vi "sendDefaultILCOutputs.vi"(8 "error in (no error)":errorcluster, 11 "Model in":refnum<class "Model.lvclass">) -> (0 "error out":errorcluster, 3 "Model out":refnum<class "Model.lvclass">)   [LabVIEW 2015, in "Model.lvclass"]
uses:
  Model.lvclass
  Typedefs/Actuate Settings.ctl
  Typedefs/ControlMode.ctl
  Model.lvclass/Model.ctl
  Actuator/IActuator/IActuator.lvclass
  <userlib>/Common/ILC/ILC/ILC.lvclass
  Typedefs/FAMTTypedefs.lvlib
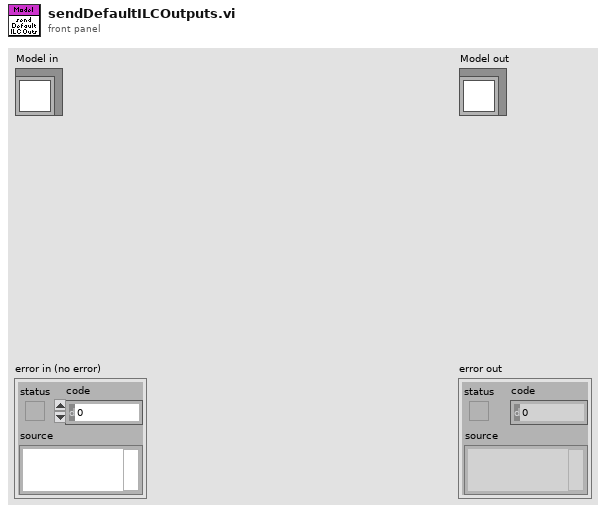
[diagram p1: front panel]
types:
  T1 = typedef "FAMTTypedefs.lvlib/ControlMode.ctl" = enum16{"PSV", "FCV", "Both"}
  T2 = typedef "FAMTTypedefs.lvlib/Actuate Settings.ctl" = cluster{"Control Mode":T1, "Control Value":dbl, "Measured Value":dbl[unit], "FCV Value":dbl}
  T3 = typedef "FAMTTypedefs.lvlib/Flow Control Settings.ctl" = cluster{"DAC Channel":u8, "ROT Bias":u8, "Minimum Voltage":dbl, "Maximum Voltage":dbl, "Off Value":dbl}
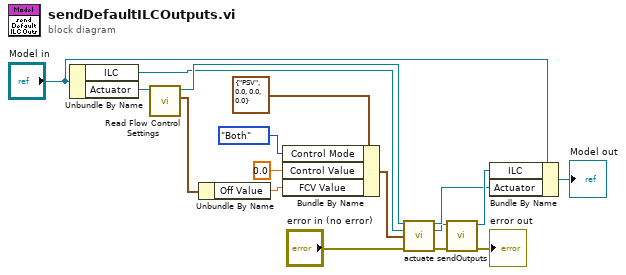
[diagram p0: block diagram]
diagram:
  n1 = Unbundle By Name("Model in") -> ("ILC"=w10:refnum<class "ILC.lvclass">, "Actuator"=w1:refnum<class "IActuator.lvclass">)
  n2 = call-dynamic "Read Flow Control Settings.vi"("IActuator in"=w1) -> ("Flow Control Settings"=w14:T3, "IActuator out"=w13:refnum<class "IActuator.lvclass">)  [unwired: 9 in]
  n3 = Unbundle By Name(w14) -> ("Off Value"=w3:dbl)
  n4 = Bundle By Name(cluster=T2 {"Control Mode"=enum."PSV", "Control Value"=0.0, "Measured Value"=0.0, "FCV Value"=0.0} ("Actuate Settings"), "Control Mode"=ControlMode."Both", "Control Value"=0.0, "FCV Value"=w3) -> (w5:T2)
  n5 = call-dynamic "actuate.vi"("IActuator in"=w13, "ILC in"=w10, "Actuate Settings"=w5, "error in (no error)"="error in (no error)") -> ("IActuator out"=w12:refnum<class "IActuator.lvclass">, "ILC out"=w11:refnum<class "ILC.lvclass">, "error out"=w8:errorcluster)  [unwired: 9 in]
  n6 = call <userlib>:"sendOutputs.vi"("error in (no error)"=w8, "ILC in"=w11) -> ("error out"=→"error out":errorcluster, "ILC out"=w16:refnum<class "ILC.lvclass">)  [unwired: 8 in]
  n7 = Bundle By Name(cluster="Model in", "ILC"=w16, "Actuator"=w12) -> (→"Model out":refnum<class "Model.lvclass">)
